vi "Circurit_Builder.vi"(3 "error in (no error)":errorcluster, 5 "Data in":string) -> (0 "error out (no error)":errorcluster, 2 "DataOut":string)   [LabVIEW 2011]
doc: "This VI connects components between two or more nodes. It also checks for differeintial connections.\n\nExample 1: Connect component 1 on card 1 --> following string: 1 1\nExample 2: Connect component 2 & 5 on card 3 --> following string: 3 18\nExample 3: Disconnect all components from card 2 --> following string: 2 0"
uses:
  Server_Globals.vi
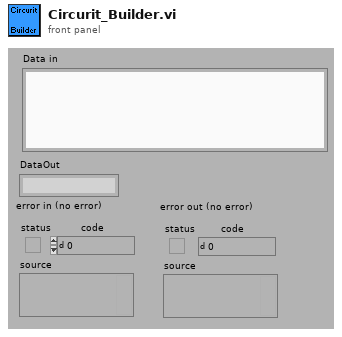
[diagram p1: front panel]
types:
  T1 = cluster{"I/O Settings":u64[], "Instrument Handle":cluster{"5402":refnum<k15>, " 5112":refnum<k15>, "4072":refnum<k15>, "USB":refnum<visa-resource-name>, "4110":refnum<k15>}, "Logfile":refnum<file>, "Log Level":i8, "Clear":i32[], "OS Set":cluster{"instrument handle out":refnum<k15>, "remaining string":string, "Settings":cluster{"Horizontal Conf.":cluster{"Min. Sample rate":dbl, "Reference position":dbl, "Record Length":i16}, "Channel A":cluster{"Enable":bool, "Vertical coupling":dbl, "Vertical range":dbl, "Vertical offset":dbl, "Probe attenuation":dbl}, "Channel B":cluster{"Enable":bool, "Vertical coupling":dbl, "Vertical range":dbl, "Vertical offset":dbl, "Probe attenuation":dbl}, "Trigger":cluster{"Source":enum8{"channel 1", "channel 2", "Imediate", "External trigger"}, "Slope":enum8{"Positive", "Negative"}, "Coupling":enum8{"AC", "DC"}, "Level":dbl, "Holdoff":dbl, "Delay":dbl, " Timeout":dbl, " Mode":enum8{"Normal", "Auto", "Auto Level"}}, "Measurements":cluster{"Measurement 1, Channel":enum8{"Channel 1", "Channel 2", "Channel 3", "Channel 4"}, "Measurement 1, Selection":u16, "Measurement 2, Channel":enum8{"Channel 1", "Channel 2", "Channel 3", "Channel 4"}, "Measurement 2,  Selection":u16, "Measurement 3, Channel":enum8{"Channel 1", "Channel 2", "Channel 3", "Channel 4"}, "Measurement 3, Selection 3":u16}}}, "DC Power Supply":cluster{"0":refnum<k15>, "1":refnum<k15>, "2":refnum<k15>, "3":refnum<k15>, "4":refnum<k15>}, "USB Interface":cluster{"0":refnum<visa-resource-name>, "1":refnum<visa-resource-name>, "2":refnum<visa-resource-name>, "3":refnum<visa-resource-name>, "4":refnum<visa-resource-name>}, "Function Generator":cluster{"0":refnum<k15>, "1":refnum<k15>, "2":refnum<k15>, "3":refnum<k15>, "4":refnum<k15>}, "Digital Multimeter":cluster{"0":refnum<k15>, "1":refnum<k15>, "2":refnum<k15>, "3":refnum<k15>, "4":refnum<k15>}, "Digital Osciliscope":cluster{"0":refnum<k15>, "1":refnum<k15>, "2":refnum<k15>, "3":refnum<k15>, "4":refnum<k15>}, "To M Server":string, "Adres":string[][], "Matrix version":string, "MD5":string, "Digital Multimeter Card 2":cluster{"0":string, "1":string, "2":string, "3":string, "4":string}}
  T2 = cluster{"0":string, "1":string, "2":string, "3":string, "4":string}
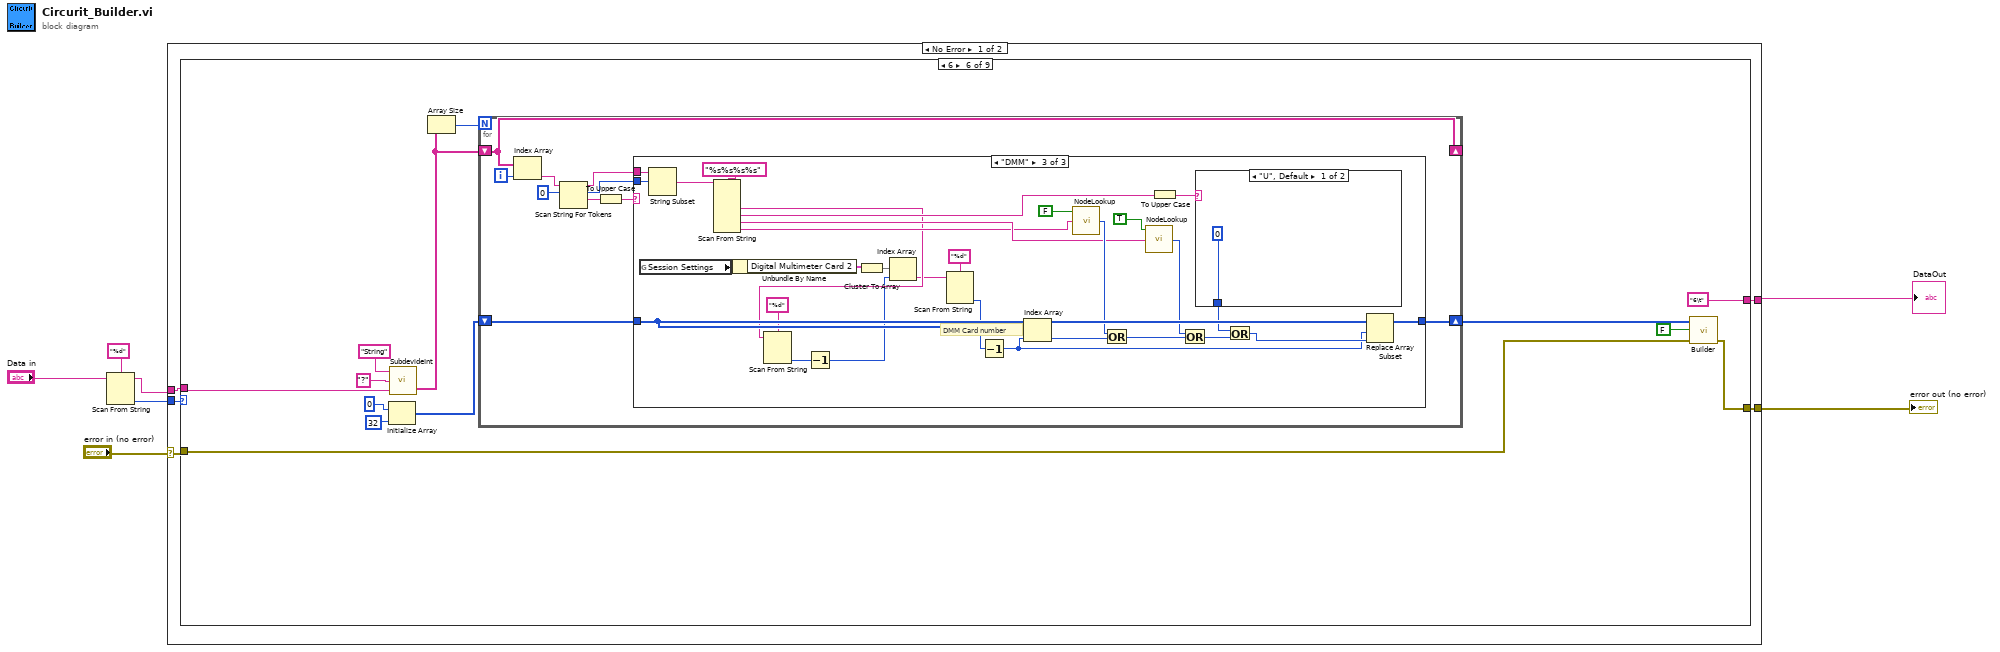
[diagram p0: block diagram]
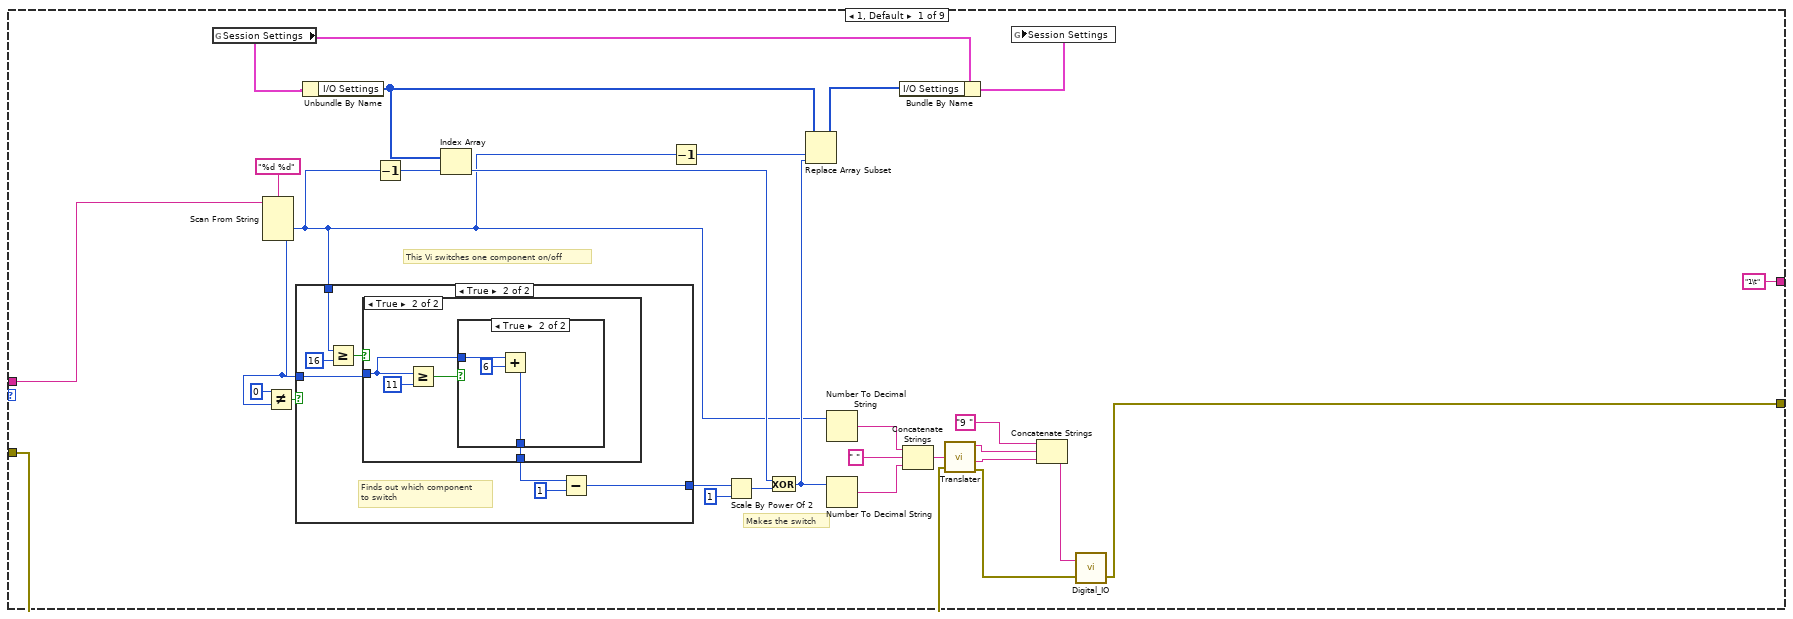
[diagram p2: hidden frame]
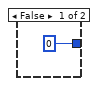
[diagram p3: hidden frame]
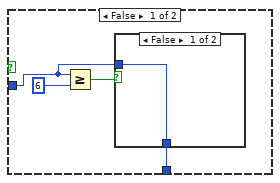
[diagram p4: hidden frame]
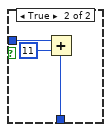
[diagram p5: hidden frame]
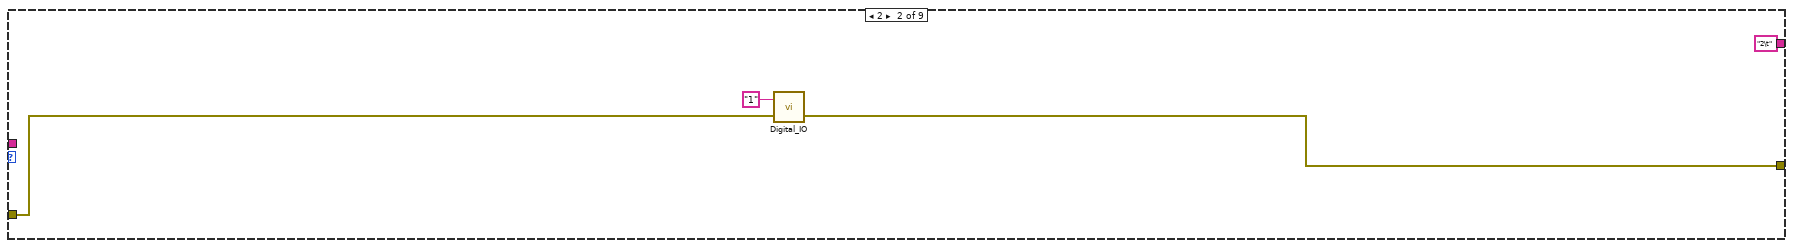
[diagram p7: hidden frame]
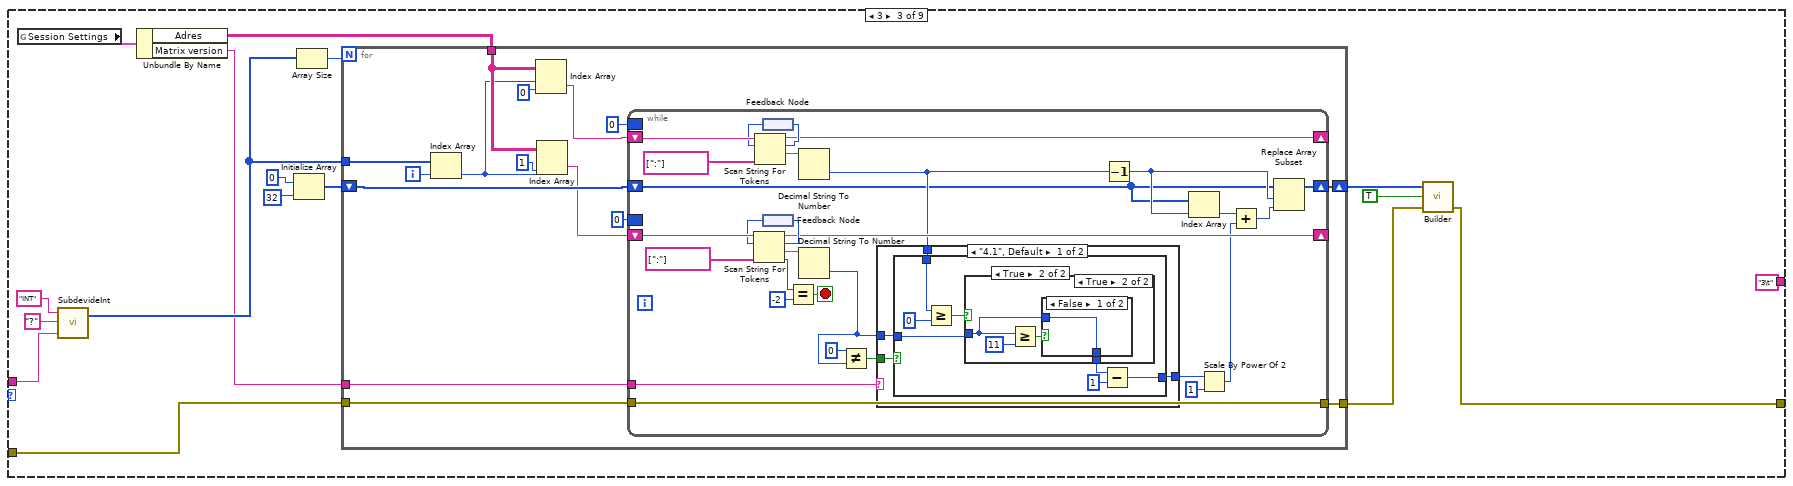
[diagram p8: hidden frame]
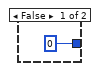
[diagram p9: hidden frame]
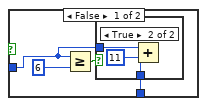
[diagram p10: hidden frame]
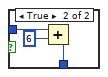
[diagram p12: hidden frame]
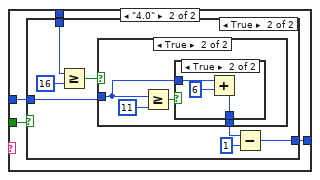
[diagram p13: hidden frame]
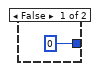
[diagram p14: hidden frame]
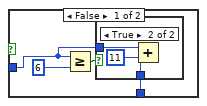
[diagram p15: hidden frame]
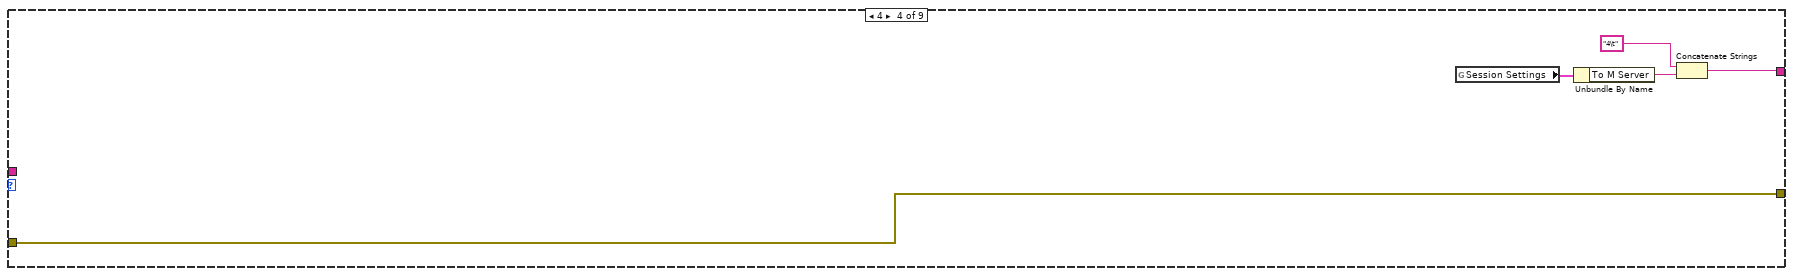
[diagram p18: hidden frame]
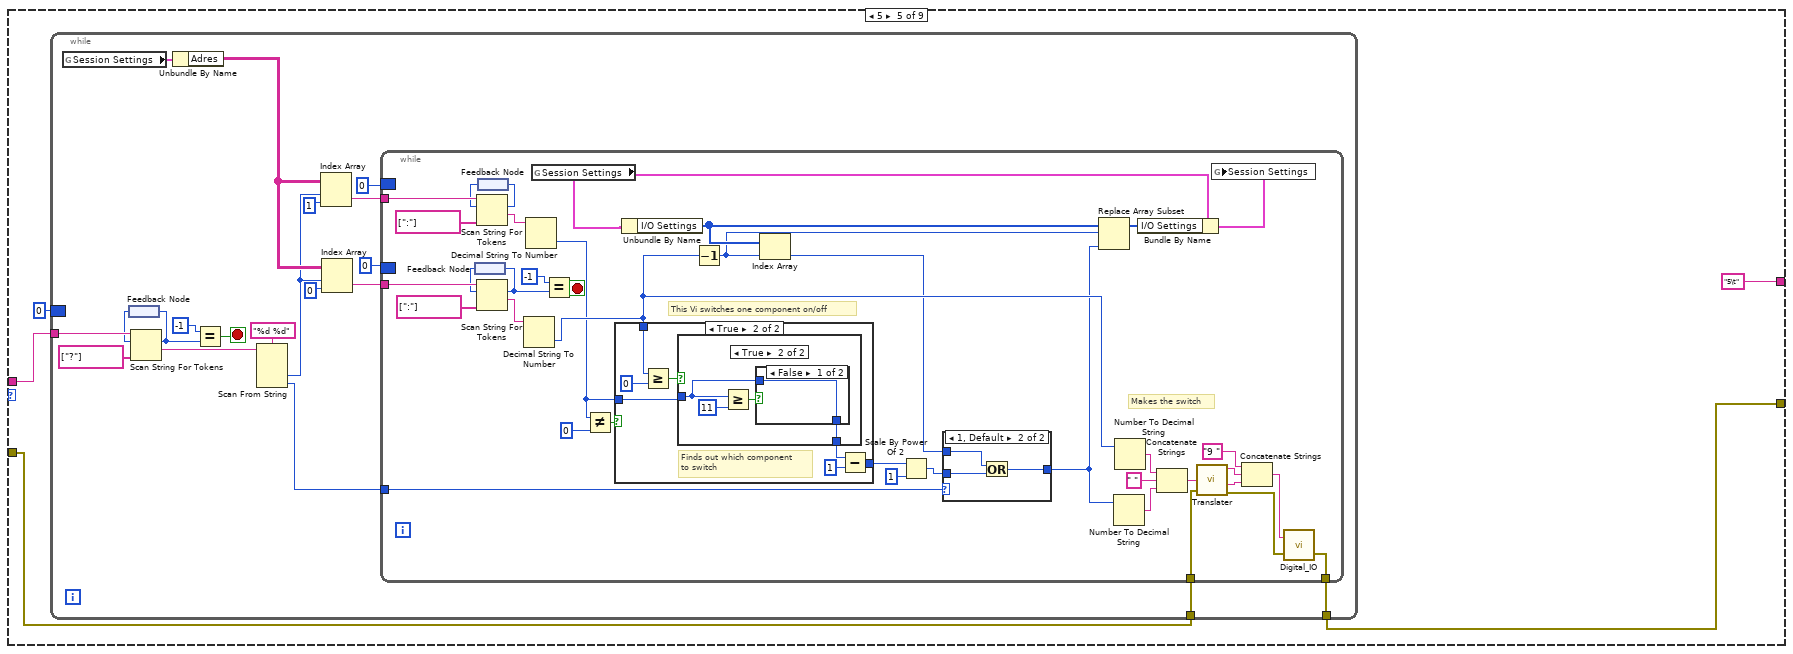
[diagram p19: hidden frame]
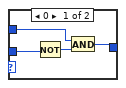
[diagram p20: hidden frame]
diagram:
  n1 = Scan From String(format string="%d", input string="Data in") -> (remaining string=w2:string, output 1=w4:i32)  [unwired: 3 in, 2 out]
  n2 = case shown="No Error" "error in (no error)" {
    selector: "error in (no error)" -> [w9 w521]
    tunnel: [w12 w521] -> w7
    tunnel: [w11 ""] -> w6
    tunnel: w4 -> [w10 _]
    tunnel: w2 -> [w8 _]
    frame No Error {
      n3 = case shown="6" w10 {
        tunnel: w9 -> [w14 w69 w83 w187 w192 w296 w374 w427 w441]
        tunnel: [w17 w68 w81 w187 w194 w295 w373 w427 w436] -> w12
        tunnel: ["1\t" "2\t" "3\t" w188 "5\t" "6\t" "7\t" w429 w435] -> w11
        tunnel: w8 -> [w15 _ w78 _ w195 w298 w380 w425 w432]
        frame 1, Default {
          # "This Vi switches one component on/off"
          # "Makes the switch"
          n4 = global read "Server_Globals.vi" "Session Settings"() -> (w37:T1)
          n5 = Scan From String(format string="%d %d", input string=w15) -> (output 1=w18:i32, output 2=w32:i32)  [unwired: 4 in, 3 out]
          n6 = Not Equal?(x=0, y=w32) -> (x != y?=w35:bool)
          n7 = case shown="True" w35 {
            tunnel: w32 -> [_ w46]
            tunnel: w18 -> [_ w48]
            tunnel: [0 w43] -> w22
            frame False {
            }
            frame True {
              # "Finds out which component\nto switch"
              n8 = Greater Or Equal?(x=w48, y=16) -> (x >= y?=w47:bool)
              n9 = case shown="True" w47 {
                tunnel: w46 -> [w51 w59]
                tunnel: [w50 w58] -> w45
                frame False {
                  n10 = Greater Or Equal?(x=w51, y=6) -> (x >= y?=w53:bool)
                  n11 = case shown="False" w53 {
                    tunnel: w51 -> [w54 w57]
                    tunnel: [w54 w55] -> w50
                    frame False {
                    }
                    frame True {
                      n12 = Add(x=w57, y=11) -> (x+y=w55:i32)
                    }
                  }
                }
                frame True {
                  n13 = Greater Or Equal?(x=w59, y=11) -> (x >= y?=w60:bool)
                  n14 = case shown="True" w60 {
                    tunnel: w59 -> [w62 w65]
                    tunnel: [w62 w63] -> w58
                    frame False {
                    }
                    frame True {
                      n15 = Add(x=w65, y=6) -> (x+y=w63:i32)
                    }
                  }
                }
              }
              n16 = Subtract(x=w45, y=1) -> (x-y=w43:i32)
            }
          }
          n17 = Unbundle By Name(w37) -> ("I/O Settings"=w40:u64[])
          n18 = Decrement(x=w18) -> (x-1=w20:i32)
          n19 = Index Array(array=w40, index=w20) -> (element=w34:u64)
          n20 = Decrement(x=w18) -> (x-1=w19:i32)
          n21 = Scale By Power Of 2(n=w22, x=1) -> (x*2^n=w23:i32)
          n22 = Exclusive Or(1:w23, 2:w34) -> (0:w30:u64)
          n23 = Replace Array Subset(array=w40, new element=w30, index=w19) -> (w39:u64[])
          n24 = Number To Decimal String(number=w18) -> (decimal integer string=w26:string)  [unwired: 1 in]
          n25 = Number To Decimal String(number=w30) -> (decimal integer string=w25:string)  [unwired: 1 in]
          n26 = Bundle By Name(cluster=w37, "I/O Settings"=w39) -> (w38:T1)
          n27 = Concatenate Strings(w26, " ", w25) -> (w27:string)
          n28 = call "Translater.vi"("In"=w27, "error in (no error)"=w14) -> ("Card"=w29:string, "Comp"=w28:string, "error out (no error)"=w13:errorcluster)  [unwired: 2 in]
          n29 = global write "Server_Globals.vi" "Session Settings"(w38) -> ()
          n30 = Concatenate Strings("9 ", w29, w28) -> (w33:string)
          n31 = call "Digital_IO.vi"("error in"=w13, "Data in"=w33) -> ("error out (no error)"=w17:errorcluster)  [unwired: 1 in]
        }
        frame 2 {
          n32 = call "Digital_IO.vi"("error in"=w69, "Data in"="1") -> ("error out (no error)"=w68:errorcluster)  [unwired: 1 in]
        }
        frame 3 {
          n33 = global read "Server_Globals.vi" "Session Settings"() -> (w85:T1)
          n34 = call "SubdevideInt.vi"("Input String"=w78, "Delimiter"="?", "INT or String"="INT") -> ("Output Array"=w77:i32[])  [unwired: 1 out]
          n35 = Unbundle By Name(w85) -> ("Adres"=w84:string[][], "Matrix version"=w70:string)
          n36 = Initialize Array(0, 32) -> (w74:i32[])
          n37 = Array Size(array=w77) -> (size(s)=w73:i32)
          n38 = for {
            N: w73 -> [_]
            tunnel: w84 -> [w95]
            tunnel: w77 -> [w94]
            shift-right: [w90] -> w80
            shift-left: w74 -> [w99]
            tunnel: w83 -> [w88]
            tunnel: [w89] -> w82
            tunnel: w70 -> [w87]
            i -> [w91]
            n39 = Index Array(array=w94, index=w91) -> (element=w93:i32)
            n40 = Index Array(array=w95, index (row)=w93, index (col)=0) -> (element=w98:string)
            n41 = Index Array(array=w95, index (row)=w93, index (col)=1) -> (element=w96:string)
            n42 = while {
              shift-right: [w122] -> _
              shift-left: w98 -> [w130]
              shift-right: [w121] -> _
              shift-left: w96 -> [w129]
              shift-right: [w104] -> w90
              shift-left: w99 -> [w108]
              tunnel: [w103] -> w89
              tunnel: w88 -> [w103]
              border: 0 -> [_]
              border: 0 -> [_]
              tunnel: w87 -> [w102]
              stop <- w118 stop-if-true
              n43 = feedback #1() -> (w125:i32)
              n44 = Scan String For Tokens(6:string[] [":"], 8:w125, 9:w130) -> (1:w117:string, 2:w126:i32, 3:w122:string)  [unwired: 3 in, 1 out]
              n45 = feedback-in #1(w126) -> ()
              n46 = feedback #2() -> (w123:i32)
              n47 = Scan String For Tokens(6:string[] [":"], 8:w123, 9:w129) -> (0:w120:i32, 1:w116:string, 2:w124:i32, 3:w121:string)  [unwired: 3 in]
              n48 = feedback-in #2(w124) -> ()
              n49 = Equal?(x=w120, y=-2) -> (x = y?=w118:bool)
              n50 = Decimal String To Number(string=w117) -> (number=w110:i32)  [unwired: 2 in, 1 out]
              n51 = Decimal String To Number(string=w116) -> (number=w113:i32)  [unwired: 2 in, 1 out]
              n52 = Not Equal?(x=0, y=w113) -> (x != y?=w114:bool)
              n53 = case shown="\"4.1\", Default" w102 {
                tunnel: w114 -> [w131 w162]
                tunnel: w113 -> [w134 w161]
                tunnel: [w132 w160] -> w111
                tunnel: w110 -> [w133 w159]
                frame "4.1", Default {
                  n54 = case shown="True" w131 {
                    tunnel: w134 -> [_ w139]
                    tunnel: w133 -> [_ w141]
                    tunnel: [0 w136] -> w132
                    frame False {
                    }
                    frame True {
                      n55 = Greater Or Equal?(x=w141, y=0) -> (x >= y?=w140:bool)
                      n56 = case shown="True" w140 {
                        tunnel: w139 -> [w144 w152]
                        tunnel: [w143 w151] -> w138
                        frame False {
                          n57 = Greater Or Equal?(x=w144, y=6) -> (x >= y?=w146:bool)
                          n58 = case shown="True" w146 {
                            tunnel: w144 -> [w147 w150]
                            tunnel: [w147 w148] -> w143
                            frame False {
                            }
                            frame True {
                              n59 = Add(x=w150, y=11) -> (x+y=w148:i32)
                            }
                          }
                        }
                        frame True {
                          n60 = Greater Or Equal?(x=w152, y=11) -> (x >= y?=w153:bool)
                          n61 = case shown="False" w153 {
                            tunnel: w152 -> [w155 w158]
                            tunnel: [w155 w156] -> w151
                            frame False {
                            }
                            frame True {
                              n62 = Add(x=w158, y=6) -> (x+y=w156:i32)
                            }
                          }
                        }
                      }
                      n63 = Subtract(x=w138, y=1) -> (x-y=w136:i32)
                    }
                  }
                }
                frame "4.0" {
                  n64 = case shown="True" w162 {
                    tunnel: w161 -> [_ w167]
                    tunnel: w159 -> [_ w169]
                    tunnel: [0 w164] -> w160
                    frame False {
                    }
                    frame True {
                      n65 = Greater Or Equal?(x=w169, y=16) -> (x >= y?=w168:bool)
                      n66 = case shown="True" w168 {
                        tunnel: w167 -> [w172 w180]
                        tunnel: [w171 w179] -> w166
                        frame False {
                          n67 = Greater Or Equal?(x=w172, y=6) -> (x >= y?=w174:bool)
                          n68 = case shown="True" w174 {
                            tunnel: w172 -> [w175 w178]
                            tunnel: [w175 w176] -> w171
                            frame False {
                            }
                            frame True {
                              n69 = Add(x=w178, y=11) -> (x+y=w176:i32)
                            }
                          }
                        }
                        frame True {
                          n70 = Greater Or Equal?(x=w180, y=11) -> (x >= y?=w181:bool)
                          n71 = case shown="True" w181 {
                            tunnel: w180 -> [w183 w186]
                            tunnel: [w183 w184] -> w179
                            frame False {
                            }
                            frame True {
                              n72 = Add(x=w186, y=6) -> (x+y=w184:i32)
                            }
                          }
                        }
                      }
                      n73 = Subtract(x=w166, y=1) -> (x-y=w164:i32)
                    }
                  }
                }
              }
              n74 = Decrement(x=w110) -> (x-1=w109:i32)
              n75 = Index Array(array=w108, index=w109) -> (element=w107:i32)
              n76 = Scale By Power Of 2(n=w111, x=1) -> (x*2^n=w106:i32)
              n77 = Add(x=w107, y=w106) -> (x+y=w105:i32)
              n78 = Replace Array Subset(array=w108, new element=w105, index=w109) -> (w104:i32[])
            }
          }
          n79 = call "Builder.vi"("error in (no error)"=w82, "Clear Cards"=TRUE, "Array IN"=w80) -> ("error out (no error)"=w81:errorcluster)  [unwired: 2 in]
        }
        frame 4 {
          n80 = global read "Server_Globals.vi" "Session Settings"() -> (w191:T1)
          n81 = Unbundle By Name(w191) -> ("To M Server"=w189:string)
          n82 = Concatenate Strings("4\t", w189) -> (w188:string)
        }
        frame 5 {
          n83 = while {
            tunnel: w195 -> [w215]
            tunnel: [w201] -> w194
            border: 0 -> [_]
            tunnel: w192 -> [w197]
            stop <- w212 stop-if-true
            n84 = global read "Server_Globals.vi" "Session Settings"() -> (w211:T1)
            n85 = feedback #3() -> (w200:i32)
            n86 = Scan String For Tokens(6:string[] ["?"], 8:w200, 9:w215) -> (1:w214:string, 2:w199:i32)  [unwired: 3 in, 2 out]
            n87 = feedback-in #3(w199) -> ()
            n88 = Unbundle By Name(w211) -> ("Adres"=w208:string[][])
            n89 = Equal?(x=-1, y=w199) -> (x = y?=w212:bool)
            n90 = Scan From String(format string="%d %d", input string=w214) -> (output 1=w207:i32, output 2=w198:i32)  [unwired: 4 in, 3 out]
            n91 = Index Array(array=w208, index (row)=w207, index (col)=1) -> (element=w205:string)
            n92 = Index Array(array=w208, index (row)=w207, index (col)=0) -> (element=w209:string)
            n93 = while {
              tunnel: w209 -> [w251]
              tunnel: w205 -> [w253]
              tunnel: [w231] -> w201
              tunnel: w198 -> [w225]
              border: 0 -> [_]
              border: 0 -> [_]
              tunnel: w197 -> [w218]
              stop <- w249 stop-if-true
              # "Makes the switch"
              # "This Vi switches one component on/off"
              n94 = feedback #4() -> (w247:i32)
              n95 = Scan String For Tokens(6:string[] [":"], 8:w247, 9:w251) -> (1:w248:string, 2:w246:i32)  [unwired: 3 in, 2 out]
              n96 = feedback-in #4(w246) -> ()
              n97 = feedback #5() -> (w244:i32)
              n98 = Scan String For Tokens(6:string[] [":"], 8:w244, 9:w253) -> (1:w228:string, 2:w245:i32)  [unwired: 3 in, 2 out]
              n99 = feedback-in #5(w245) -> ()
              n100 = Decimal String To Number(string=w248) -> (number=w230:i32)  [unwired: 2 in, 1 out]
              n101 = Decimal String To Number(string=w228) -> (number=w220:i32)  [unwired: 2 in, 1 out]
              n102 = global read "Server_Globals.vi" "Session Settings"() -> (w240:T1)
              n103 = Equal?(x=-1, y=w246) -> (x = y?=w249:bool)
              n104 = Not Equal?(x=w220, y=0) -> (x != y?=w239:bool)
              n105 = case shown="True" w239 {
                tunnel: w220 -> [_ w266]
                tunnel: w230 -> [_ w268]
                tunnel: [0 w263] -> w226
                frame False {
                }
                frame True {
                  # "Finds out which component\nto switch"
                  n106 = Greater Or Equal?(x=w268, y=0) -> (x >= y?=w267:bool)
                  n107 = case shown="True" w267 {
                    tunnel: w266 -> [w271 w279]
                    tunnel: [w270 w278] -> w265
                    frame False {
                      n108 = Greater Or Equal?(x=w271, y=7) -> (x >= y?=w273:bool)
                      n109 = case shown="True" w273 {
                        tunnel: w271 -> [w274 w277]
                        tunnel: [w274 w275] -> w270
                        frame False {
                        }
                        frame True {
                          n110 = Add(x=w277, y=11) -> (x+y=w275:i32)
                        }
                      }
                    }
                    frame True {
                      n111 = Greater Or Equal?(x=w279, y=11) -> (x >= y?=w280:bool)
                      n112 = case shown="False" w280 {
                        tunnel: w279 -> [w282 w285]
                        tunnel: [w282 w283] -> w278
                        frame False {
                        }
                        frame True {
                          n113 = Add(x=w285, y=6) -> (x+y=w283:i32)
                        }
                      }
                    }
                  }
                  n114 = Subtract(x=w265, y=1) -> (x-y=w263:i32)
                }
              }
              n115 = Unbundle By Name(w240) -> ("I/O Settings"=w243:u64[])
              n116 = Decrement(x=w230) -> (x-1=w229:i32)
              n117 = Index Array(array=w243, index=w229) -> (element=w224:u64)
              n118 = Scale By Power Of 2(n=w226, x=1) -> (x*2^n=w223:i32)
              n119 = case shown="1, Default" w225 {
                tunnel: w224 -> [w256 w261]
                tunnel: w223 -> [w257 w260]
                tunnel: [w255 w259] -> w221
                frame 0 {
                  n120 = Not(x=w257) -> (.not. x?=w258:i32)
                  n121 = And(x=w256, y=w258) -> (x .and. y?=w255:u64)
                }
                frame 1, Default {
                  n122 = Or(x=w261, y=w260) -> (x .or. y?=w259:u64)
                }
              }
              n123 = Replace Array Subset(array=w243, new element=w221, index=w229) -> (w242:u64[])
              n124 = Number To Decimal String(number=w221) -> (decimal integer string=w222:string)  [unwired: 1 in]
              n125 = Number To Decimal String(number=w230) -> (decimal integer string=w233:string)  [unwired: 1 in]
              n126 = Bundle By Name(cluster=w240, "I/O Settings"=w242) -> (w241:T1)
              n127 = Concatenate Strings(w233, " ", w222) -> (w234:string)
              n128 = call "Translater.vi"("In"=w234, "error in (no error)"=w218) -> ("Card"=w236:string, "Comp"=w235:string, "error out (no error)"=w217:errorcluster)  [unwired: 2 in]
              n129 = global write "Server_Globals.vi" "Session Settings"(w241) -> ()
              n130 = Concatenate Strings("9 ", w236, w235) -> (w238:string)
              n131 = call "Digital_IO.vi"("error in"=w217, "Data in"=w238) -> ("error out (no error)"=w231:errorcluster)  [unwired: 1 in]
            }
          }
        }
        frame 6 {
          n132 = Initialize Array(i64 0, 32) -> (w289:i64[])
          n133 = call "SubdevideInt.vi"("Input String"=w298, "Delimiter"="?", "INT or String"="String") -> ("Output Array"=w291:string[])  [unwired: 1 out]
          n134 = Array Size(array=w291) -> (size(s)=w292:i32)
          n135 = for {
            N: w292 -> [_]
            shift-right: [w301] -> _
            shift-left: w291 -> [w301]
            shift-right: [w299] -> w287
            shift-left: w289 -> [w300]
            i -> [w308]
            n136 = Index Array(array=w301, index=w308) -> (element=w307:string)
            n137 = Scan String For Tokens(8:0, 9:w307) -> (1:w304:string, 2:w302:i32, 3:w303:string)  [unwired: 4 in, 1 out]
            n138 = To Upper Case(1:w304) -> (0:w305:string)
            n139 = case shown="\"DMM\"" w305 {
              tunnel: w303 -> [w320 _ w352]
              tunnel: w302 -> [w323 _ w351]
              tunnel: w300 -> [w319 w324 w349]
              tunnel: [w318 w324 w348] -> w299
              frame "OSC" {
                # "OSC Card number"
                n140 = String Subset(string=w320, offset (0)=w323) -> (substring=w322:string)  [unwired: 1 in]
                n141 = Scan From String(format string="%s%s%s", input string=w322) -> (output 2=w313:string, output 3=w315:string)  [unwired: 6 in, 3 out]
                n142 = Equal?(x="2", y=w313) -> (x = y?=w314:bool)
                n143 = Decrement(x=16) -> (x-1=w309:i32)
                n144 = call "NodeLookup.vi"("String"=w315, "Boolean"=w314) -> ("Numeric"=w311:i32)  [unwired: 3 in]
                n145 = Index Array(array=w319, index=w309) -> (element=w316:i64)
                n146 = Or(x=w311, y=w316) -> (x .or. y?=w317:i64)
                n147 = Replace Array Subset(array=w319, new element=w317, index=w309) -> (w318:i64[])
              }
              frame Default {
              }
              frame "DMM" {
                # "DMM Card number"
                n148 = global read "Server_Globals.vi" "Session Settings"() -> (w332:T1)
                n149 = String Subset(string=w352, offset (0)=w351) -> (substring=w354:string)  [unwired: 1 in]
                n150 = Scan From String(format string="%s%s%s%s", input string=w354) -> (output 1=w330:string, output 2=w341:string, output 3=w336:string, output 4=w335:string)  [unwired: 6 in, 3 out]
                n151 = Unbundle By Name(w332) -> ("Digital Multimeter Card 2"=w333:T2)
                n152 = Scan From String(format string="%d", input string=w330) -> (output 1=w329:i32)  [unwired: 3 in, 3 out]
                n153 = Decrement(x=w329) -> (x-1=w328:i32)
                n154 = Cluster To Array(cluster=w333) -> (array=w334:string[])
                n155 = Index Array(array=w334, index=w328) -> (element=w326:string)
                n156 = Scan From String(format string="%d", input string=w326) -> (output 1=w325:i32)  [unwired: 3 in, 3 out]
                n157 = Decrement(x=w325) -> (x-1=w337:i32)
                n158 = Index Array(array=w349, index=w337) -> (element=w350:i64)
                n159 = call "NodeLookup.vi"("String"=w335, "Boolean"=FALSE) -> ("Numeric"=w346:i32)  [unwired: 3 in]
                n160 = Or(x=w346, y=w350) -> (x .or. y?=w345:i64)
                n161 = call "NodeLookup.vi"("String"=w336, "Boolean"=TRUE) -> ("Numeric"=w343:i32)  [unwired: 3 in]
                n162 = To Upper Case(1:w341) -> (0:w342:string)
                n163 = Or(x=w343, y=w345) -> (x .or. y?=w340:i64)
                n164 = case shown="\"U\", Default" w342 {
                  tunnel: [0 w357] -> w338
                  frame "U", Default {
                  }
                  frame "I" {
                    w356 = 21
                    n165 = Greater Or Equal?(x=w356, y=11) -> (x >= y?=w360:bool)
                    n166 = case shown="True" w360 {
                      tunnel: w356 -> [w364 w367]
                      tunnel: [w364 w365] -> w363
                      frame False {
                      }
                      frame True {
                        n167 = Add(x=w367, y=6) -> (x+y=w365:i32)
                      }
                    }
                    n168 = Subtract(x=w363, y=1) -> (x-y=w358:i32)
                    n169 = Scale By Power Of 2(n=w358, x=1) -> (x*2^n=w357:i32)
                  }
                }
                n170 = Or(x=w338, y=w340) -> (x .or. y?=w339:i64)
                n171 = Replace Array Subset(array=w349, new element=w339, index=w337) -> (w348:i64[])
              }
            }
          }
          n172 = call "Builder.vi"("error in (no error)"=w296, "Clear Cards"=FALSE, "Array IN"=w287) -> ("error out (no error)"=w295:errorcluster)  [unwired: 2 in]
        }
        frame 7 {
          n173 = call <vilib>:"Space Constant.vi"() -> ("String"=w371:string)
          n174 = call "SubdevideInt.vi"("Input String"=w380, "Delimiter"=w371, "INT or String"="INT") -> ("Output Array"=w379:i32[])  [unwired: 1 out]
          n175 = Index Array(array=w379, index=1) -> (element=w368:i32)
          n176 = Index Array(array=w379, index=0) -> (element=w372:i32)
          n177 = Add(x=w368, y=128) -> (x+y=w375:i32)
          n178 = Greater Or Equal?(x=w368, y=0) -> (x >= y?=w369:bool)
          n179 = case shown="True" w369 {
            tunnel: w375 -> [_ w404]
            tunnel: w374 -> [w386 w398]
            tunnel: [w385 w397] -> w373
            tunnel: w372 -> [_ w394]
            tunnel: w368 -> [w387 _]
            frame False {
              n180 = Number To Decimal String(number=w387) -> (decimal integer string=w388:string)  [unwired: 1 in]
              n181 = Concatenate Strings("Enterd value is: ", w388) -> (w384:string)
              n182 = Bundle By Name(cluster=w386, "status"=TRUE, "source"=w384) -> (w385:errorcluster)
            }
            frame True {
              w416 = "9 "  # Set Card Data
              # "Finds the card nr"
              n183 = global read "Server_Globals.vi" "Session Settings"() -> (w412:T1)
              n184 = Unbundle By Name(w412) -> ("I/O Settings"=w411:u64[], "Adres"=w395:string[][])
              n185 = Index Array(array=w395, index (row)=w394, index (col)=0) -> (element=w392:string)
              n186 = Scan String For Tokens(6:string[] [":"], 9:w392) -> (3:w391:string)  [unwired: 4 in, 3 out]
              n187 = Decimal String To Number(string=w391) -> (number=w390:i32)  [unwired: 2 in, 1 out]
              n188 = Decrement(x=w390) -> (x-1=w407:i32)
              n189 = Index Array(array=w411, index=w407) -> (element=w406:u64)
              n190 = Number To Decimal String(number=w406) -> (decimal integer string=w408:string)  [unwired: 1 in]
              n191 = Number To Decimal String(number=w390) -> (decimal integer string=w409:string)  [unwired: 1 in]
              n192 = call <vilib>:"Space Constant.vi"() -> ("String"=w410:string)
              n193 = Concatenate Strings(w409, w410, w408) -> (w405:string)
              n194 = call "Translater.vi"("In"=w405, "error in (no error)"=w398) -> ("Card"=w415:string, "Comp"=w414:string, "error out (no error)"=w413:errorcluster)  [unwired: 2 in]
              n195 = Number To Decimal String(number=w404) -> (decimal integer string=w402:string)  [unwired: 1 in]
              n196 = Concatenate Strings(w416, w415, w414) -> (w403:string)
              n197 = Replace Substring(2:3, 3:11, 4:w402, 5:w403) -> (1:w399:string)  [unwired: 1 out]
              n198 = call "Digital_IO.vi"("error in"=w413, "Data in"=w399) -> ("error out (no error)"=w397:errorcluster)  [unwired: 1 in]
            }
          }
        }
        frame 8 {
          n199 = global read "Server_Globals.vi" "Session Settings"() -> (w431:T1)
          n200 = Unbundle By Name(w431) -> ("MD5"=w426:string)
          n201 = String Length(string=w425) -> (length=w424:i32)
          n202 = String Length(string=w426) -> (length=w423:i32)
          n203 = Equal?(x=w424, y=w423) -> (x = y?=w421:bool)
          n204 = call "Boolean2String.vi"("input 1"=w421) -> ("resulting string"=w420:string)  [unwired: 4 in]
          n205 = call <vilib>:"Space Constant.vi"() -> ("String"=w419:string)
          n206 = Concatenate Strings("\"TEST\" MD5 sum = 32 ", w420, w419) -> (w417:string)
          n207 = Equal?(x=w426, y=w425) -> (x = y?=w428:bool)
          n208 = call "Boolean2String.vi"("input 1"=w428) -> ("resulting string"=w422:string)  [unwired: 4 in]
          n209 = Concatenate Strings("8\t", w417, w422) -> (w429:string)
        }
        frame 0 {
          # "Writing the new circuit to the matrix"
          # "Setting which cards to clear\nCards with a 1 in the clear varible should not be cleared"
          # "Comparing the circuit all ready build in the matrix"
          n210 = call "Subdevide.vi"("Input String"=w432, "Delimiter"="?") -> ("Output Array"=w433:string[])
          n211 = Array Size(array=w433) -> (size(s)=w439:i32)
          n212 = for {
            N: w439 -> [_]
            tunnel: w433 -> [w465] mode=indexing
            shift-right: [w477] -> w440
            shift-left: w441 -> [w478]
            tunnel: [w466] -> w437 mode=indexing
            # "All cards involved in the circuit are marked with a 1"
            n213 = global read "Server_Globals.vi" "Session Settings"() -> (w474:T1)
            n214 = Scan From String(format string="%d %d", input string=w465) -> (output 1=w475:i32, output 2=w473:i32)  [unwired: 4 in, 3 out]
            n215 = Decrement(x=w475) -> (x-1=w472:i32)
            n216 = Unbundle By Name(w474) -> ("Clear"=w467:i32[], "I/O Settings"=w468:u64[])
            n217 = Index Array(array=w468, index=w472) -> (element=w480:u64)
            n218 = Equal?(x=w480, y=w473) -> (x = y?=w479:bool)
            n219 = case "Check if component already connected/disconnected" shown="False" w479 {
              tunnel: w468 -> [w486 w490]
              tunnel: [w487 w490] -> w469
              tunnel: w473 -> [w484 _]
              tunnel: w472 -> [w485 _]
              tunnel: w478 -> [w483 w489]
              tunnel: [w483 w489] -> w477
              tunnel: [w482 ""] -> w466
              tunnel: w465 -> [w482 _]
              frame False {
                n220 = Replace Array Subset(array=w486, new element=w484, index=w485) -> (w487:u64[])
              }
              frame True {
              }
            }
            n221 = Replace Array Subset(array=w467, new element=1, index=w472) -> (w470:i32[])
            n222 = Bundle By Name(cluster=w474, "Clear"=w470, "I/O Settings"=w469) -> (w481:T1)
            n223 = global write "Server_Globals.vi" "Session Settings"(w481) -> ()
          }
          n224 = case shown="No Error" w440 {
            selector: w440 -> [w499 w520]
            tunnel: [w498 w520] -> w434
            frame No Error {
              n225 = global read "Server_Globals.vi" "Session Settings"() -> (w501:T1)
              n226 = Unbundle By Name(w501) -> ("Clear"=w497:i32[], "I/O Settings"=w491:u64[])
              n227 = for {
                tunnel: w497 -> [w512] mode=indexing
                shift-right: [w509] -> w494
                shift-left: "3 " -> [w510]
                tunnel: [0] -> w500 mode=indexing
                tunnel: w491 -> [w506] mode=indexing
                i -> [w511]
                n228 = Equal?(x=0, y=w512) -> (x = y?=w504:bool)
                n229 = Not Equal?(x=w506, y=0) -> (x != y?=w505:bool)
                n230 = And(x=w504, y=w505) -> (x .and. y?=w503:bool)
                n231 = case shown="False" w503 {
                  tunnel: w511 -> [_ w517]
                  tunnel: w510 -> [w514 w519]
                  tunnel: [w514 w518] -> w509
                  frame False {
                  }
                  frame True {
                    n232 = Number To Decimal String(number=w517) -> (decimal integer string=w516:string)  [unwired: 1 in]
                    n233 = Concatenate Strings(w519, w516, ",") -> (w518:string)
                  }
                }
              }
              n234 = Bundle By Name(cluster=w501, "Clear"=w500) -> (w502:T1)
              n235 = String Length(string=w494) -> (length=w493:i32)
              n236 = Decrement(x=w493) -> (x-1=w492:i32)
              n237 = global write "Server_Globals.vi" "Session Settings"(w502) -> ()
              n238 = String Subset(string=w494, length (rest)=w492) -> (substring=w495:string)  [unwired: 1 in]
              n239 = call "Digital_IO.vi"("error in"=w499, "Data in"=w495) -> ("error out (no error)"=w498:errorcluster)  [unwired: 1 in]
            }
            frame Error {
            }
          }
          n240 = case shown="No Error" w434 {
            selector: w434 -> [w442 w464]
            tunnel: w437 -> [w444 _]
            tunnel: [w443 w464] -> w436
            tunnel: ["0\t" ""] -> w435
            frame No Error {
              n241 = Array Size(array=w444) -> (size(s)=w445:i32)
              n242 = for {
                N: w445 -> [_]
                tunnel: w444 -> [w453]
                tunnel: [w452] -> w443
                tunnel: w442 -> [w451]
                i -> [w450]
                n243 = Index Array(array=w453, index=w450) -> (element=w448:string)
                n244 = Not Equal?(x="", y=w448) -> (x != y?=w449:bool)
                n245 = case shown="True" w449 {
                  tunnel: w448 -> [_ w458]
                  tunnel: [w454 w457] -> w452
                  tunnel: w451 -> [w454 w456]
                  frame False {
                  }
                  frame True {
                    w462 = "9 "  # Set Card Data
                    n246 = call "Translater.vi"("In"=w458, "error in (no error)"=w456) -> ("Card"=w460:string, "Comp"=w459:string, "error out (no error)"=w455:errorcluster)  [unwired: 2 in]
                    n247 = Concatenate Strings(w462, w460, w459) -> (w461:string)
                    n248 = call "Digital_IO.vi"("error in"=w455, "Data in"=w461) -> ("error out (no error)"=w457:errorcluster)  [unwired: 1 in]
                  }
                }
              }
            }
            frame Error {
            }
          }
        }
      }
    }
    frame Error {
    }
  }
  "error out (no error)" <- w7
  "DataOut" <- w6
